vi "Delete Pump.vi"(5 "pump cmd array":T2[](array[typedef]), 7 "Pump updates":T1[](array[typedef]) {"Update Time" format="%.2f"}, 8 "Timeout":u32=120, 9 "write interval (s)":dbl=5.0, 10 "Time":dbl format="%.2f", 11 "VISA":refnum<visa-resource-name>) -> (2 "Pump updates out":T1[](array[typedef]) {"Update Time" format="%.2f"}, 3 "pump cmd array out":T2[](array[typedef]))   [LabVIEW 2019]
uses:
  Pump updates.ctl
  pump 2 flows.ctl
  modbusrtu/SerialParameters.ctl
  modbusrtu/MB Serial Master Query Write Single Register (poly).vi
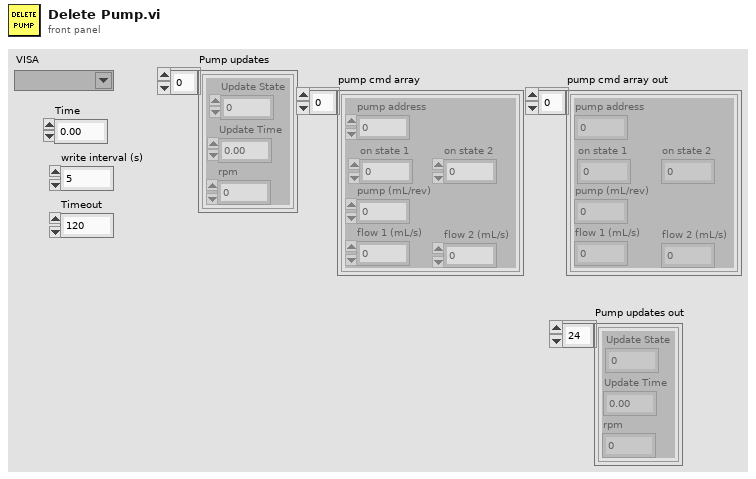
[diagram p1: front panel]
types:
  T1 = typedef "Pump updates.ctl" = cluster{"Update State":i16, "Update Time":dbl, "rpm":dbl}
  T2 = typedef "pump 2 flows.ctl" = cluster{"pump address":u8, "on state 1":i32, "on state 2":i32, "pump (mL/rev)":dbl, "flow 1 (mL/s)":dbl, "flow 2 (mL/s)":dbl}
  T3 = typedef "SerialParameters.ctl" = cluster{"Mode":enum16{"RTU", "ASCII"}, "Address":u16, "Address bytes":enum16{"1 byte", "2 bytes"}}
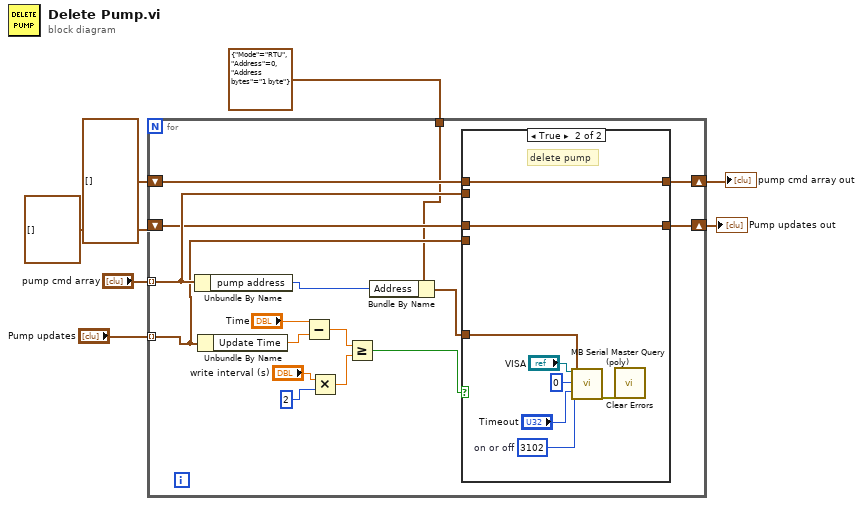
[diagram p0: block diagram]
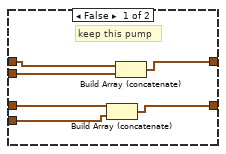
[diagram p2: hidden frame]
diagram:
  n1 = for {
    tunnel: "Pump updates" -> [w11] mode=indexing
    tunnel: "pump cmd array" -> [w14] mode=indexing
    shift-right: [w12] -> w5
    shift-left: T2[] [] -> [w13]
    shift-right: [w10] -> w4
    shift-left: T1[] [] -> [w9]
    tunnel: T3 {"Mode"=enum."RTU", "Address"=0, "Address bytes"=enum."1 byte"} ("Serial Parameters") -> [w8]
    n2 = Unbundle By Name(w14) -> ("pump address"=w16:u8)
    n3 = Unbundle By Name(w11) -> ("Update Time"=w22:dbl)
    n4 = Subtract(x="Time", y=w22) -> (x-y=w19:dbl)
    n5 = Multiply(x="write interval (s)", y=2) -> (x*y=w18:dbl)
    n6 = Greater Or Equal?(x=w19, y=w18) -> (x >= y?=w15:bool)
    n7 = Bundle By Name(cluster=w8, "Address"=w16) -> (w17:T3)
    n8 = case shown="True" w15 {
      tunnel: w17 -> [_ w30]
      tunnel: w14 -> [w29 _]
      tunnel: w13 -> [w28 w33]
      tunnel: [w27 w33] -> w12
      tunnel: w11 -> [w25 _]
      tunnel: [w24 w32] -> w10
      tunnel: w9 -> [w26 w32]
      frame False {
        # "keep this pump"
        n9 = Build Array (concatenate)(w26, w25) -> (w24:T1[])
        n10 = Build Array (concatenate)(w28, w29) -> (w27:T2[])
      }
      frame True {
        w37 = u16 3102  # on or off
        # "delete pump"
        n11 = call-poly "MB Serial Master Query (poly).vi"("VISA resource name"="VISA", "Address"=w37, "Holding Register"=u16 0, "Timeout"="Timeout", "Serial Parameters"=w30) -> ("error out"=w31:errorcluster)  [unwired: 12 in, 2 out]
        n12 = call <vilib>:"Clear Errors.vi"("error in (no error)"=w31) -> ()  [unwired: 5 in, 2 out]
      }
    }
  }
  "pump cmd array out" <- w5
  "Pump updates out" <- w4
